vi "BasicClassDocumentation_Interface.vi"(9 "EventsIn":T1, 10 "Events":T2) -> ()   [LabVIEW 2014, in "BasicClassDocumentation.lvlib" / "BasicClassDocumentation.lvclass"]
uses:
  BasicClassDocumentation.lvclass
  Framework/_Plugins/_LVCMPlugin/GCMPlugin_EventsOut.ctl
  Framework/_Plugins/_LVCMPlugin/GCMPlugin_EventsIn.ctl
  Utilites/ClassBannerEditor/ClassBannerEditor/ClassBannerEditor.xctl
  <vilib>/LabVIEW Icon API/lv_icon/Classes/Icon/Icon.lvclass
  InterfaceState.ctl
  <vilib>/LabVIEW Icon API/LabVIEW Icon API.lvlib
  Framework/_Plugins/GCMPlugin/GCMPlugin.lvclass
panel:
  in  "Apply banner color to class wire":bool=TRUE
  in  "ApplyBanner":bool
  in  "Banner":refnum<class "Icon.lvclass">(xcontrol)
  in  "Localized Name":string
  out "Icon":picture
  in  "Description":string
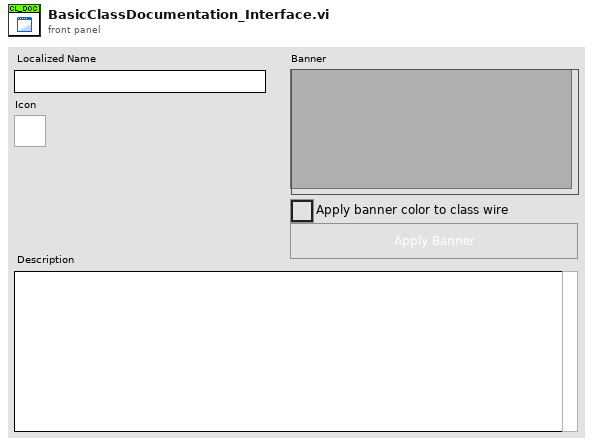
[diagram p1: front panel]
types:
  T1 = typedef "GCMPlugin.lvclass/GCMPlugin_EventsIn.ctl" = cluster{"Stop":refnum<user-event>, "ItemSelected":refnum<user-event>, "ItemDeselected":refnum<user-event>, "PluginActivated":refnum<user-event>, "PluginDeactivated":refnum<user-event>}
  T2 = typedef "GCMPlugin.lvclass/GCMPlugin_EventsOut.ctl" = cluster{"ItemEdited":refnum<user-event>}
  T3 = typedef "BasicClassDocumentation.lvlib/BasicClassDocumentation.lvclass/InterfaceState.ctl" = enum16{"Initialize", "WaitForEvent", "RunIconEditor"}
  T4 = typedef "imagedata.ctl" = cluster{"image type":i32, "image depth":i32, "image":u8[], "mask":u8[], "colors":u32[], "Rectangle":cluster{"left":i16, "top":i16, "right":i16, "bottom":i16}}
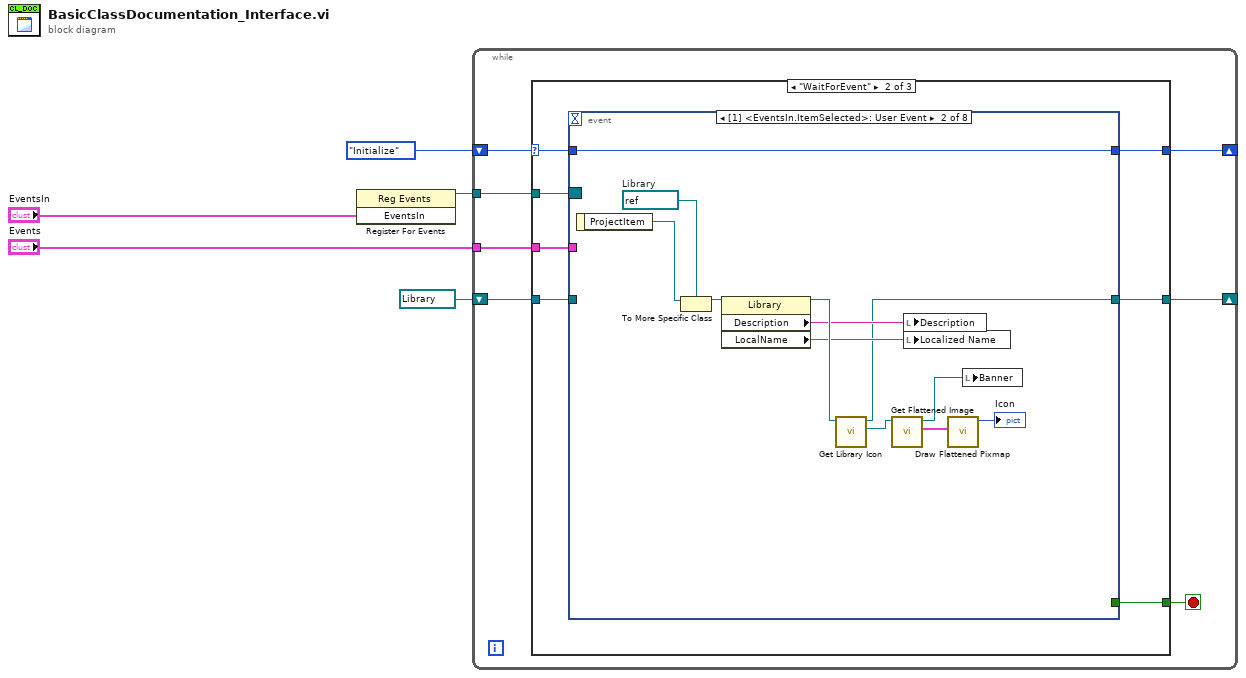
[diagram p0: block diagram]
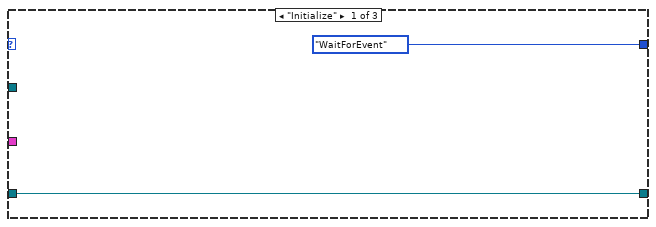
[diagram p2: hidden frame]
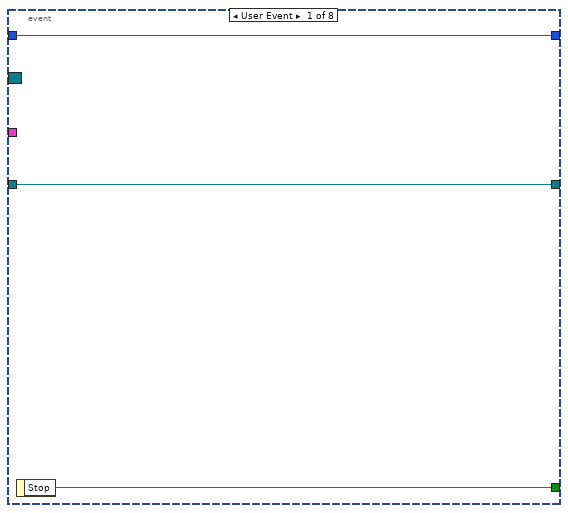
[diagram p3: hidden frame]
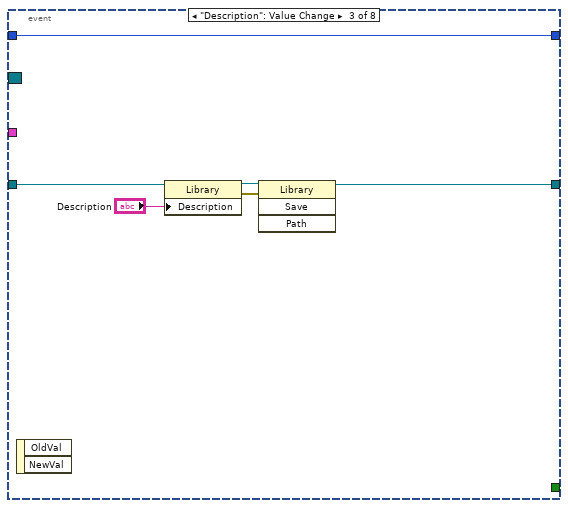
[diagram p4: hidden frame]
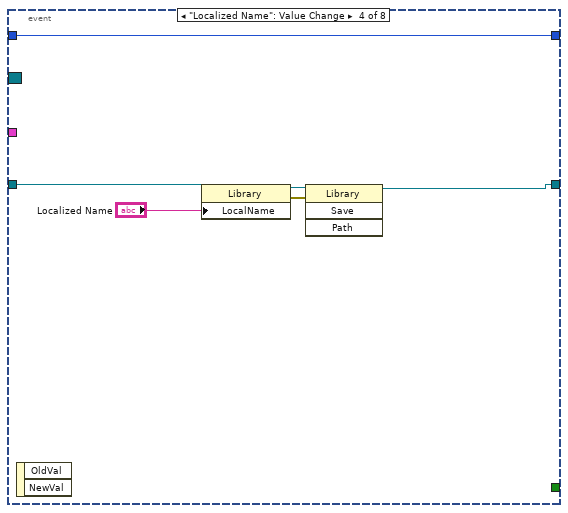
[diagram p5: hidden frame]
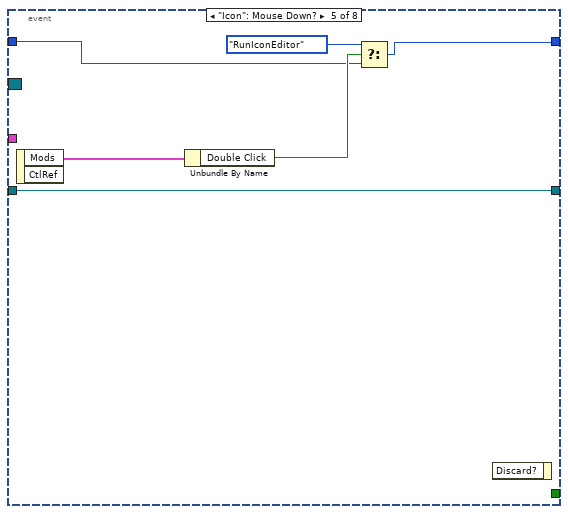
[diagram p6: hidden frame]
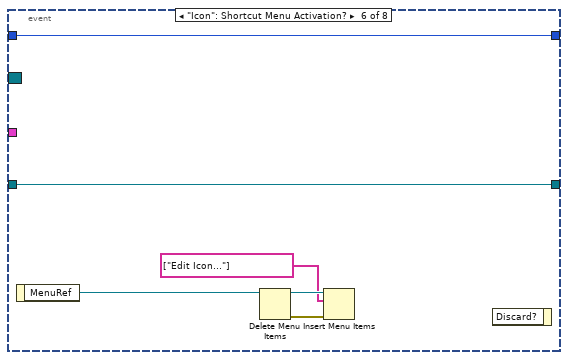
[diagram p7: hidden frame]
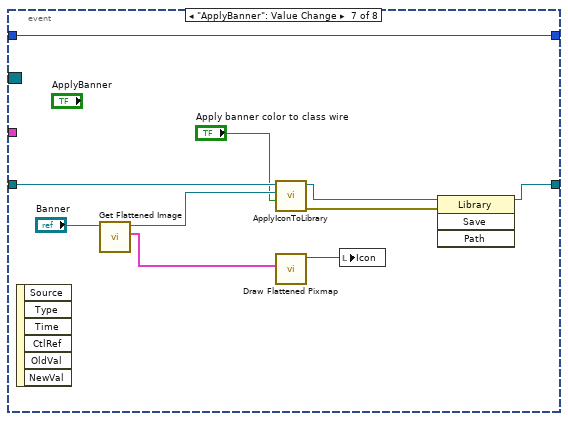
[diagram p8: hidden frame]
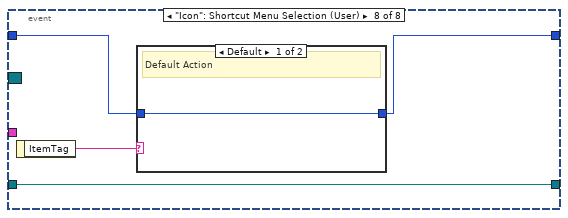
[diagram p9: hidden frame]
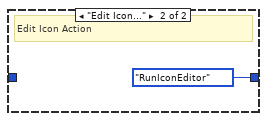
[diagram p10: hidden frame]
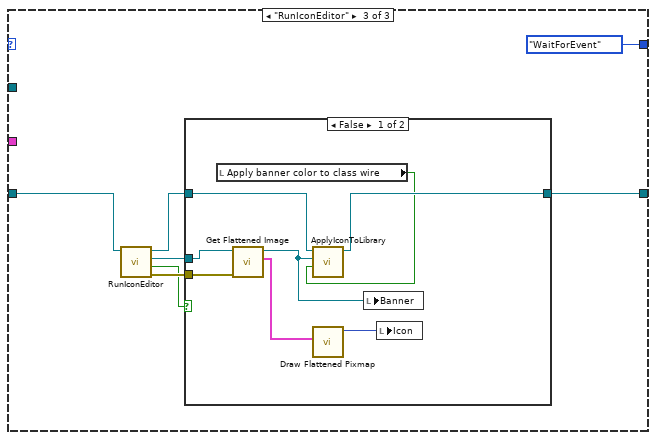
[diagram p11: hidden frame]
diagram:
  n1 = register-events("EventsIn") -> (reference out=w4:refnum<event-registration>)  [unwired: 2 in, 1 out]
  n2 = while {
    tunnel: w4 -> [w12]
    tunnel: "Events" -> [w11]
    shift-right: [w8] -> _
    shift-left: refnum<vi> refnum ("Library Refnum out") -> [w9]
    shift-right: [w6] -> _
    shift-left: InterfaceState."Initialize" ("State") -> [w7]
    stop <- w10 stop-if-true
    n3 = case shown="\"WaitForEvent\"" w7 {
      selector: w7 -> [_ w16 _]
      tunnel: w12 -> [_ w21 _]
      tunnel: w11 -> [_ w20 _]
      tunnel: [_ w19 _] -> w10
      tunnel: w9 -> [w13 w18 w79]
      tunnel: [w13 w17 w78] -> w8
      tunnel: [InterfaceState."WaitForEvent" ("State") w15 InterfaceState."WaitForEvent" ("State")] -> w6
      frame "Initialize" {
      }
      frame "WaitForEvent" {
        n4 = event shown="[1] <EventsIn.ItemSelected>: User Event" {
          selector: w21 -> [_ _ _ _ _ _ _ _]
          dyn-events: _ -> [_ _ _ _ _ _ _ _]
          timeout: _ -> [_ _ _ _ _ _ _ _]
          tunnel: w20 -> [_ _ _ _ _ _ _ _]
          tunnel: [w24 _ _ _ _ _ _ _] -> w19
          tunnel: w18 -> [w23 _ w42 w48 w53 w56 w69 w71]
          tunnel: [w23 w28 w38 w44 w53 w56 w66 w71] -> w17
          tunnel: w16 -> [w22 w25 w37 w43 w51 w55 w70 w72]
          tunnel: [w22 w25 w37 w43 w49 w55 w70 w73] -> w15
          event User Event {
            n5 = event-data() -> ("Stop"=w24:bool)  [unwired: 1 in]
          }
          event User Event {
            w29 = refnum<vi> refnum  # Library
            n6 = event-data() -> ("ProjectItem"=w27:refnum<vi>)  [unwired: 1 in]
            n7 = To More Specific Class(target class=w29, reference=w27) -> (specific class reference=w33:refnum<vi>)  [unwired: 1 in, 1 out]
            n8 = property class="Library"(reference=w33) -> (reference out=w35:refnum<vi>, "Description"=w30:string, "LocalName"=w34:string)  [unwired: 1 in, 1 out]
            n9 = call <vilib>:"Get Library Icon.vi"("Library Refnum in"=w35) -> ("Icon"=w36:refnum<class "Icon.lvclass">, "Library Refnum out"=w28:refnum<vi>)  [unwired: 8 in, 1 out]
            n10 = call <vilib>:"Get Flattened Image.vi"("lv_icon.lvlib:Icon.lvclass in"=w36) -> ("Color Image"=w31:T4, "lv_icon.lvlib:Icon.lvclass out"=w26:refnum<class "Icon.lvclass">)  [unwired: 7 in, 2 out]
            n11 = local write "Description"(w30) -> ()
            n12 = local write "Localized Name"(w34) -> ()
            n13 = call <vilib>:"Draw Flattened Pixmap.vi"("image data"=w31) -> ("new picture"=→"Icon":picture)  [unwired: 8 in]
            n14 = local write "Banner"(w26) -> ()
          }
          event "Description": Value Change {
            n15 = event-data() -> ()  [unwired: 1 in, 2 out]
            n16 = property class="Library"(reference=w42, "Description"="Description") -> (reference out=w41:refnum<vi>, error out=w40:errorcluster)  [unwired: 1 in]
            n17 = invoke class="Library" method="Save"(reference=w41, error in=w40) -> (reference out=w38:refnum<vi>)  [unwired: 2 in, 3 out]
          }
          event "Localized Name": Value Change {
            n18 = event-data() -> ()  [unwired: 1 in, 2 out]
            n19 = property class="Library"(reference=w48, "LocalName"="Localized Name") -> (reference out=w47:refnum<vi>, error out=w46:errorcluster)  [unwired: 1 in]
            n20 = invoke class="Library" method="Save"(reference=w47, error in=w46) -> (reference out=w44:refnum<vi>)  [unwired: 2 in, 3 out]
          }
          event "Icon": Mouse Down? {
            n21 = event-data() -> ("Mods"=w54:cluster{"Double Click":bool, "Menu Key":bool})  [unwired: 1 in, 1 out]
            n22 = Unbundle By Name(w54) -> ("Double Click"=w52:bool)
            n23 = Select(t=InterfaceState."RunIconEditor", s=w52, f=w51) -> (s? t:f=w49:T3)
            n24 = event-data() -> ()  [unwired: 2 in, 1 out]
          }
          event "Icon": Shortcut Menu Activation? {
            n25 = event-data() -> ("MenuRef"=w57:refnum<k9>)  [unwired: 1 in]
            n26 = Delete Menu Items(9:w57) -> (0:w59:errorcluster, 3:w60:refnum<k9>)  [unwired: 3 in]
            n27 = Insert Menu Items(6:w59, 8:string[] ["Edit Icon..."] ("item names"), 9:w60) -> ()  [unwired: 3 in, 3 out]
            n28 = event-data() -> ()  [unwired: 2 in, 1 out]
          }
          event "ApplyBanner": Value Change {
            n29 = event-data() -> ()  [unwired: 1 in, 6 out]
            n30 = call <vilib>:"Get Flattened Image.vi"("lv_icon.lvlib:Icon.lvclass in"="Banner") -> ("Color Image"=w62:T4, "lv_icon.lvlib:Icon.lvclass out"=w64:refnum<class "Icon.lvclass">)  [unwired: 7 in, 2 out]
            n31 = call "ApplyIconToLibrary.vi"("Apply banner color to class wire"="Apply banner color to class wire", "Icon"=w64, "Library Refnum in"=w69) -> ("error out"=w67:errorcluster, "Library Refnum out"=w68:refnum<vi>)  [unwired: 7 in]
            n32 = call <vilib>:"Draw Flattened Pixmap.vi"("image data"=w62) -> ("new picture"=w63:picture)  [unwired: 8 in]
            n33 = local write "Icon"(w63) -> ()
            n34 = invoke class="Library" method="Save"(reference=w68, error in=w67) -> (reference out=w66:refnum<vi>)  [unwired: 2 in, 3 out]
          }
          event "Icon": Shortcut Menu Selection (User) {
            n35 = event-data() -> ("ItemTag"=w74:string)  [unwired: 1 in]
            n36 = case shown="Default" w74 {
              tunnel: [w75 InterfaceState."RunIconEditor" ("State")] -> w73
              tunnel: w72 -> [w75 _]
              frame Default {
                # "Default Action"
              }
              frame "Edit Icon..." {
                # "Edit Icon Action"
              }
            }
          }
        }
      }
      frame "RunIconEditor" {
        n37 = call "RunIconEditor.vi"("Library Refnum in"=w79) -> ("error out"=w82:errorcluster, "Canceled?"=w77:bool, "Icon out"=w80:refnum<class "Icon.lvclass">, "Library Refnum out"=w81:refnum<vi>)  [unwired: 7 in]
        n38 = case shown="False" w77 {
          tunnel: w82 -> [w89 _]
          tunnel: w81 -> [w91 w92]
          tunnel: w80 -> [w88 _]
          tunnel: [w90 w92] -> w78
          frame False {
            n39 = local read "Apply banner color to class wire"() -> (w84:bool)
            n40 = call <vilib>:"Get Flattened Image.vi"("error in (no error)"=w89, "lv_icon.lvlib:Icon.lvclass in"=w88) -> ("Color Image"=w86:T4, "lv_icon.lvlib:Icon.lvclass out"=w87:refnum<class "Icon.lvclass">)  [unwired: 6 in, 2 out]
            n41 = call "ApplyIconToLibrary.vi"("Apply banner color to class wire"=w84, "Icon"=w87, "Library Refnum in"=w91) -> ("Library Refnum out"=w90:refnum<vi>)  [unwired: 7 in, 1 out]
            n42 = call <vilib>:"Draw Flattened Pixmap.vi"("image data"=w86) -> ("new picture"=w85:picture)  [unwired: 8 in]
            n43 = local write "Banner"(w87) -> ()
            n44 = local write "Icon"(w85) -> ()
          }
          frame True {
          }
        }
      }
    }
  }
